vi "PS3 Controller.vi"(8 "error in (no error)":errorcluster, 11 "device ID":refnum<k1>) -> (0 "error out":errorcluster, 1 "Arrows":i32, 2 "Buttons control":T1, 3 "Control cluster":T2 {"Roll" scale=-1.0..1.0; "Pitch" scale=-1.0..1.0; "Vertical Speed" scale=-1.0..1.0; "Yaw Speed" scale=-1.0..1.0})   [LabVIEW 2014]
uses:
  <vilib>/Utility/inputDevices.llb/joystickAcquire.vi
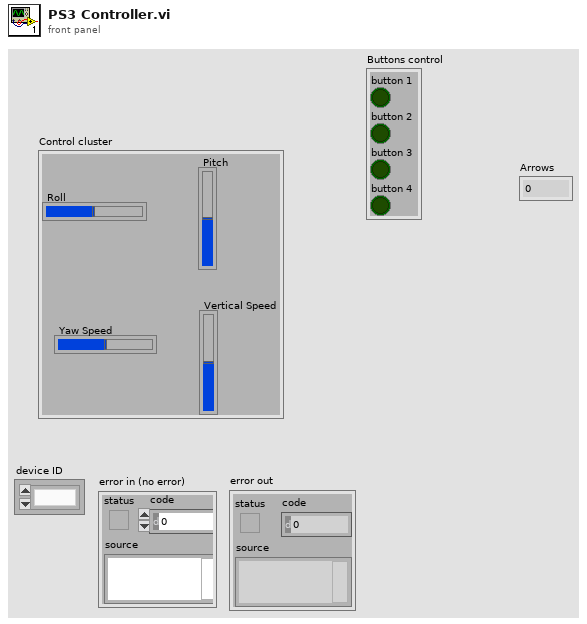
[diagram p1: front panel]
types:
  T1 = cluster{"button 1":bool, "button 2":bool, "button 3":bool, "button 4":bool}
  T2 = cluster{"Roll":dbl, "Pitch":dbl, "Vertical Speed":dbl, "Yaw Speed":dbl}
  T3 = cluster{"X axis":dbl, "Y axis":dbl, "Z axis":dbl, "X axis rotation":dbl}
  T4 = cluster{"X axis":i32, "Y axis":i32, "Z axis":i32, "X axis rotation":i32, "Y axis rotation":i32, "Z axis rotation":i32, "U axis":i32, "V axis":i32}
  T5 = cluster{"button 1":bool, "button 2":bool, "button 3":bool, "button 4":bool, "button 5":bool, "button 6":bool, "button 7":bool, "button 8":bool, "button 9":bool, "button 10":bool, "button 11":bool, "button 12":bool, "button 13":bool, "button 14":bool, "button 15":bool, "button 16":bool, "button 17":bool, "button 18":bool, "button 19":bool, "button 20":bool, "button 21":bool, "button 22":bool, "button 23":bool, "button 24":bool, "button 25":bool, "button 26":bool, "button 27":bool, "button 28":bool, "button 29":bool, "button 30":bool, "button 31":bool, "button 32":bool}
  T6 = cluster{"pov 1":i32, "pov 2":i32, "pov 3":i32, "pov 4":i32}
  T7 = cluster{"X axis":dbl, "Y axis":dbl, "Z axis":dbl, "X axis rotation":dbl, "Y axis rotation":dbl, "Z axis rotation":dbl, "U axis":dbl, "V axis":dbl}
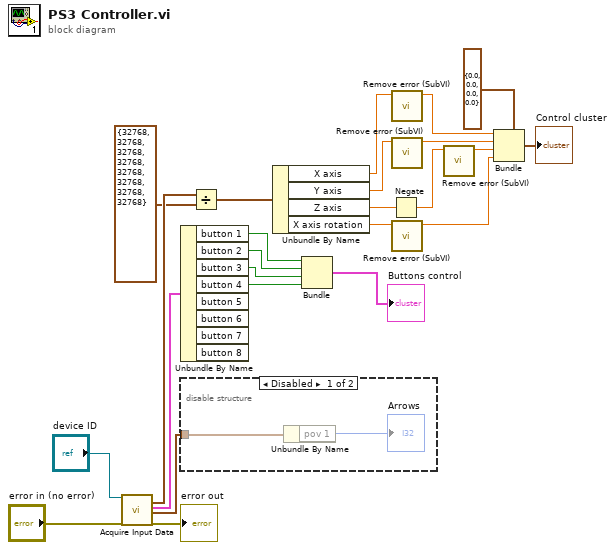
[diagram p0: block diagram]
diagram:
  n1 = call-poly <vilib>:"Acquire Input Data.vi"("device ID"="device ID", "error in (no error)"="error in (no error)") -> ("axis info"=w16:T4, "button info"=w20:T5, "direction info"=w18:T6, "error out"=→"error out":errorcluster)  [unwired: 13 in, 1 out]
  n2 = Unbundle By Name(w20) -> ("button 1"=w13:bool, "button 2"=w12:bool, "button 3"=w11:bool, "button 4"=w10:bool)  [unwired: 4 out]
  n3 = disable-structure shown="Disabled" {
    disable-tunnel: w18 -> [w25 _]
    frame Disabled {
      n4 = Unbundle By Name(w25) -> ("pov 1"=→"Arrows":i32)
    }
    frame Enabled {
    }
  }
  n5 = Divide(x=w16, y=T4 {"X axis"=32768, "Y axis"=32768, "Z axis"=32768, "X axis rotation"=32768, "Y axis rotation"=32768, "Z axis rotation"=32768, "U axis"=32768, "V axis"=32768}) -> (x/y=w17:T7)
  n6 = Unbundle By Name(w17) -> ("X axis"=w8:dbl, "Y axis"=w6:dbl, "Z axis"=w14:dbl, "X axis rotation"=w4:dbl)
  n7 = Bundle("button 1"=w13, "button 2"=w12, "button 3"=w11, "button 4"=w10) -> (→"Buttons control":T1)  [unwired: 1 in]
  n8 = Negate(x=w14) -> (-x=w5:dbl)
  n9 = call "Remove error (SubVI).vi"("X axis in"=w8) -> ("X axis out"=w7:dbl)  [unwired: 10 in]
  n10 = call "Remove error (SubVI).vi"("X axis in"=w6) -> ("X axis out"=w3:dbl)  [unwired: 10 in]
  n11 = call "Remove error (SubVI).vi"("X axis in"=w4) -> ("X axis out"=w1:dbl)  [unwired: 10 in]
  n12 = call "Remove error (SubVI).vi"("X axis in"=w5) -> ("X axis out"=w2:dbl)  [unwired: 10 in]
  n13 = Bundle(cluster=T3 {"X axis"=0.0, "Y axis"=0.0, "Z axis"=0.0, "X axis rotation"=0.0}, "X axis"=w7, "Y axis"=w3, "Z axis"=w2, "X axis rotation"=w1) -> (→"Control cluster":T3)
